vi "Get Control Information.vi"(8 "error in (no error)":errorcluster, 11 "Text Ring in":refnum<class "Text Ring.lvclass">) -> (0 "error out":errorcluster, 2 "Control Information":string[][](array[string]), 3 "Text Ring out":refnum<class "Text Ring.lvclass">)   [LabVIEW 2017, in "Localization.lvlib" / "Text Ring.lvclass"]
doc: "VI for override that is supposed to do go throgh the process for each control type and pull out the information that is necessary for each control.\n\nChoose Movement Consulting, LLC"
uses:
  Text Ring.lvclass
  C:/Apps/CMC/OpenSource/Localization/Control Info/Control Info.lvclass
  Localization.lvlib
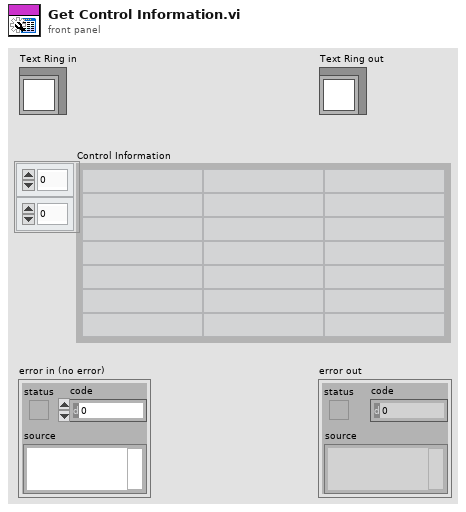
[diagram p1: front panel]
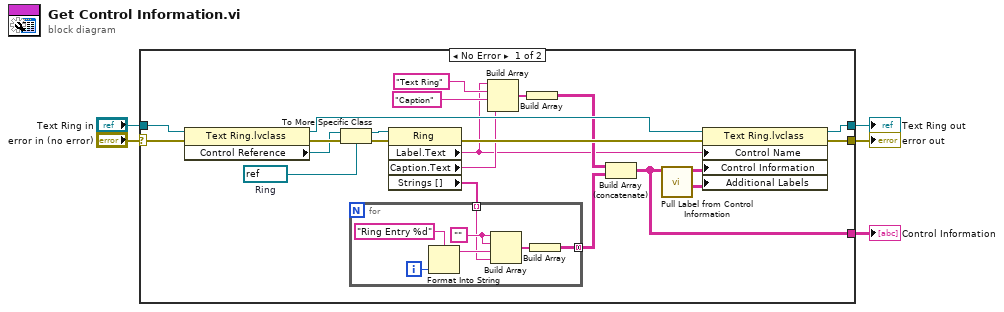
[diagram p0: block diagram]
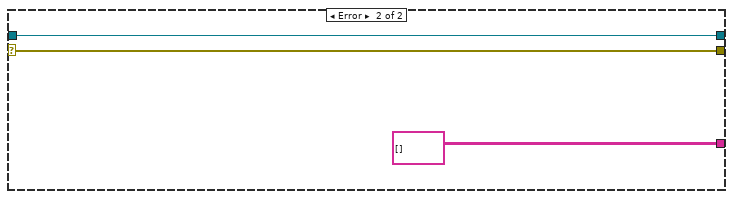
[diagram p2: hidden frame]
diagram:
  n1 = case shown="No Error" "error in (no error)" {
    selector: "error in (no error)" -> [w22 w37]
    tunnel: [w18 w37] -> w2
    tunnel: "Text Ring in" -> [w21 w36]
    tunnel: [w9 string[][] []] -> w3
    tunnel: [w16 w36] -> w1
    frame No Error {
      w27 = refnum<vi> refnum  # Ring
      n2 = property class="Text Ring.lvclass"(reference=w21, error in=w22) -> (reference out=w17:refnum<class "Text Ring.lvclass">, error out=w23:errorcluster, "Control Reference"=w20:refnum<vi>)
      n3 = To More Specific Class(target class=w27, reference=w20, error in=w23) -> (specific class reference=w26:refnum<vi>, error out=w24:errorcluster)
      n4 = property class="Ring"(reference=w26, error in=w24) -> (error out=w19:errorcluster, "Label.Text"=w6:string, "Caption.Text"=w10:string, "Strings []"=w15:string[])  [unwired: 1 out]
      n5 = for {
        tunnel: w15 -> [w28] mode=indexing
        tunnel: [w33] -> w14 mode=concatenating
        i -> [w30]
        w32 = ""
        n6 = Format Into String(format string="Ring Entry %d", w30) -> (resulting string=w29:string)  [unwired: 2 in, 1 out]
        n7 = Build Array(w32, w32, w29, w28) -> (w34:string[])
        n8 = Build Array(w34) -> (w33:string[][])
      }
      n9 = Build Array(w6, "Text Ring", "Caption", w10) -> (w25:string[])
      n10 = Build Array(w25) -> (w13:string[][])
      n11 = Build Array (concatenate)(w13, w14) -> (w9:string[][])
      n12 = call "Pull Label from Control Information.vi"("Control Caption Table"=w9) -> ("Additional Labels"=w7:string[][], "Control Information"=w8:string[][])  [unwired: 9 in]
      n13 = property class="Text Ring.lvclass"(reference=w17, error in=w19, "Control Name"=w6, "Control Information"=w8, "Additional Labels"=w7) -> (reference out=w16:refnum<class "Text Ring.lvclass">, error out=w18:errorcluster)
    }
    frame Error {
    }
  }
  "error out" <- w2
  "Text Ring out" <- w1
  "Control Information" <- w3
